vi "create server acceptor.vi"(8 "error in":errorcluster, 9 "port":u16, 11 "engine context in":refnum<class "engine context.lvclass">) -> (0 "error out":errorcluster, 3 "server acceptor out":refnum<class "server acceptor.lvclass">)   [LabVIEW 2016, in "engine context.lvclass"]
uses:
  engine context.lvclass
  connection creator/server acceptor/server acceptor.lvclass
  engine context.lvclass/engine context.ctl
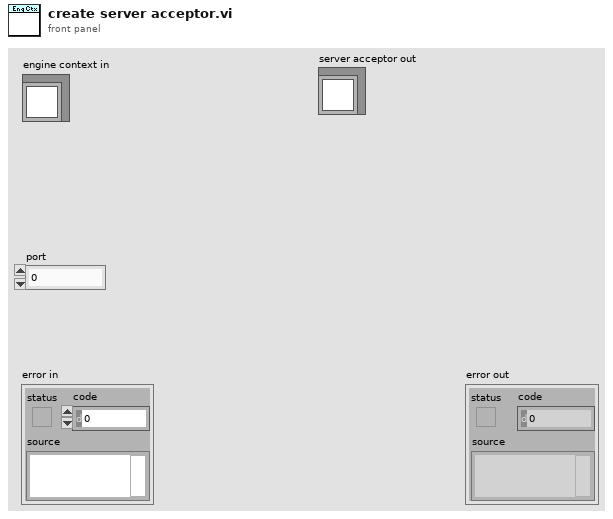
[diagram p1: front panel]
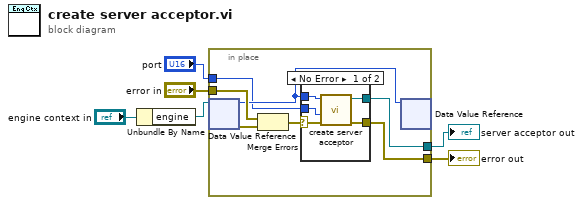
[diagram p0: block diagram]
diagram:
  n1 = Unbundle By Name("engine context in") -> ("engine"=w5:refnum<data-value>)
  n2 = in-place {
    in-place-border: "error in" -> [w13]
    in-place-border: [w10] -> w3
    in-place-border: [w9] -> w1
    in-place-border: "port" -> [w7]
    n3 = in-place-dvr #1(w5) -> (w8:u64, w12:errorcluster)
    n4 = Merge Errors(w13, w12) -> (w11:errorcluster)
    n5 = case shown="No Error" w11 {
      selector: w11 -> [w17 w19]
      tunnel: w8 -> [w18 _]
      tunnel: [w15 w19] -> w10
      tunnel: [w16 _] -> w9
      tunnel: w7 -> [w14 _]
      frame No Error {
        n6 = call "create server acceptor.vi"("error in"=w17, "port"=w14, "engine pointer"=w18) -> ("error out"=w15:errorcluster, "server acceptor out"=w16:refnum<class "server acceptor.lvclass">)  [unwired: 7 in]
      }
      frame Error {
      }
    }
    n7 = in-place-dvr #1(w8) -> ()  [unwired: 2 out]
  }
  "error out" <- w3
  "server acceptor out" <- w1
